vi "Total Heat Transfer Area.vi"(9 "NDHX Number of Tubes":dbl, 10 "NDHX Tube Length (m)":dbl, 11 "NDHX Tube Diameter (m)":dbl) -> (3 "Total Heat Transfer Area (m^2)":dbl)   [LabVIEW 2019]
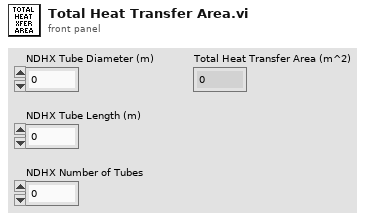
[diagram p1: front panel]
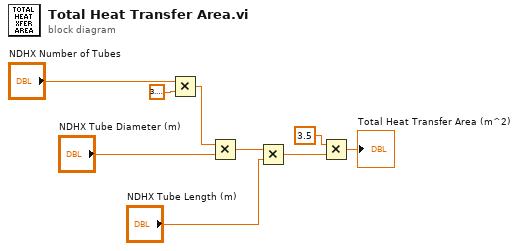
[diagram p0: block diagram]
diagram:
  n1 = Multiply(x="NDHX Number of Tubes", y=3.141592653589793) -> (x*y=w1:dbl)
  n2 = Multiply(x=w1, y="NDHX Tube Diameter (m)") -> (x*y=w5:dbl)
  n3 = Multiply(x=w5, y="NDHX Tube Length (m)") -> (x*y=w7:dbl)
  n4 = Multiply(x=3.5, y=w7) -> (x*y=→"Total Heat Transfer Area (m^2)":dbl)
